vi "Commit.vi"(8 "error in (no error)":errorcluster, 11 "Driver in":refnum<class "Driver.lvclass">) -> (0 "error out":errorcluster, 3 "Driver out":refnum<class "Driver.lvclass">)   [LabVIEW 2023, in "HAF.lvlib" / "Driver.lvclass"]
doc: "Iterates through Driver Settings for a specific Command, applying any that haven't yet been applied."
uses:
  Driver.lvclass
  DriverSetting/DriverSetting.lvclass
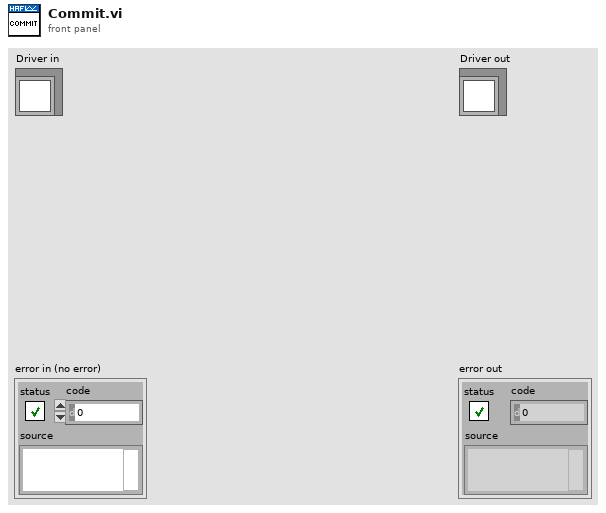
[diagram p1: front panel]
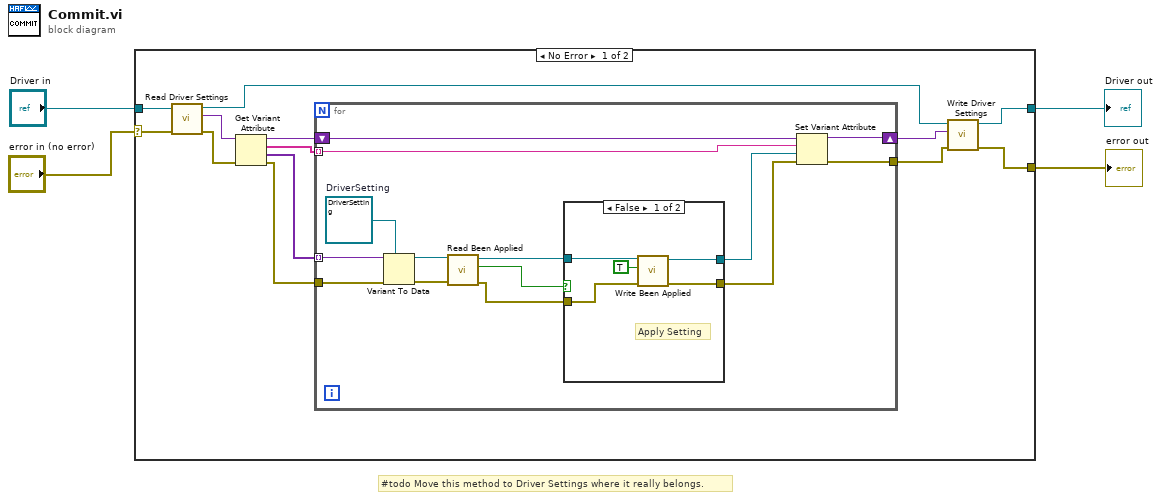
[diagram p0: block diagram]
diagram:
  # "#todo Move this method to Driver Settings where it really belongs."
  n1 = case shown="No Error" "error in (no error)" {
    selector: "error in (no error)" -> [w16 w40]
    tunnel: [w5 w40] -> w3
    tunnel: [w6 w39] -> w1
    tunnel: "Driver in" -> [w17 w39]
    frame No Error {
      n2 = call-dynamic "Read Driver Settings.vi"("error in (no error)"=w16, "Driver in"=w17) -> ("error out"=w15:errorcluster, "Driver Settings"=w14:variant, "Driver out"=w8:refnum<class "Driver.lvclass">)  [unwired: 7 in]
      n3 = Get Variant Attribute(Variant=w14, error in=w15) -> (duplicate Variant=w13:variant, names=w12:string[], values=w11:variant[], error out=w10:errorcluster)  [unwired: 2 in]
      n4 = for {
        shift-right: [w18] -> w9
        shift-left: w13 -> [w23]
        tunnel: w12 -> [w22] mode=indexing
        tunnel: w11 -> [w30] mode=indexing
        tunnel: w10 -> [w31]
        tunnel: [w19] -> w7
        w29 = refnum<class "DriverSetting.lvclass"> refnum  # DriverSetting
        n5 = Variant To Data(error in=w31, type=w29, Variant=w30) -> (data=w28:refnum<class "DriverSetting.lvclass">, error out=w27:errorcluster)
        n6 = call-dynamic "Read Been Applied.vi"("error in (no error)"=w27, "DriverSetting in"=w28) -> ("error out"=w24:errorcluster, "Been Applied"=w25:bool, "DriverSetting out"=w26:refnum<class "DriverSetting.lvclass">)  [unwired: 7 in]
        n7 = case shown="False" w25 {
          tunnel: w26 -> [w36 w38]
          tunnel: w24 -> [w34 w37]
          tunnel: [w33 w37] -> w20
          tunnel: [w32 w38] -> w21
          frame False {
            # "Apply Setting"
            n8 = call-dynamic "Write Been Applied.vi"("error in (no error)"=w34, "Been Applied"=TRUE, "DriverSetting in"=w36) -> ("error out"=w33:errorcluster, "DriverSetting out"=w32:refnum<class "DriverSetting.lvclass">)  [unwired: 7 in]
          }
          frame True {
            # "Do nothing as\nalready applied"
          }
        }
        n9 = Set Variant Attribute(Variant=w23, name=w22, value=w21, error in=w20) -> (Variant out=w18:variant, error out=w19:errorcluster)  [unwired: 1 out]
      }
      n10 = call-dynamic "Write Driver Settings.vi"("error in (no error)"=w7, "Driver Settings"=w9, "Driver in"=w8) -> ("error out"=w5:errorcluster, "Driver out"=w6:refnum<class "Driver.lvclass">)  [unwired: 7 in]
    }
    frame Error {
    }
  }
  "error out" <- w3
  "Driver out" <- w1
